vi "gugudan server.vi"() -> ()   [LabVIEW 2014]
panel:
  in  "사용설명서":bool
  out "로그인":bool
  in  "ID":string="ID"
  in  "PW":string="PW"
  in  "명령전달":bool
  in  "address":string="ip address"
  out "명령코드":i16[](array[numeric])
  out "참 거짓":string="상태창입니다."
  out "문자열":string="명령창 입니다."
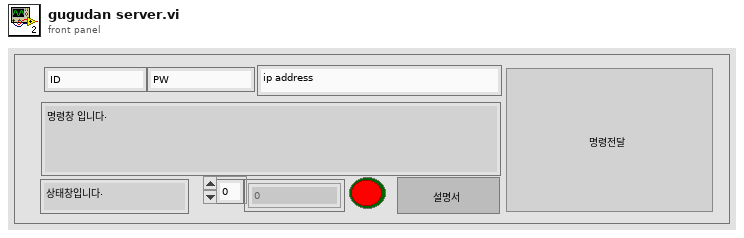
[diagram p1: front panel]
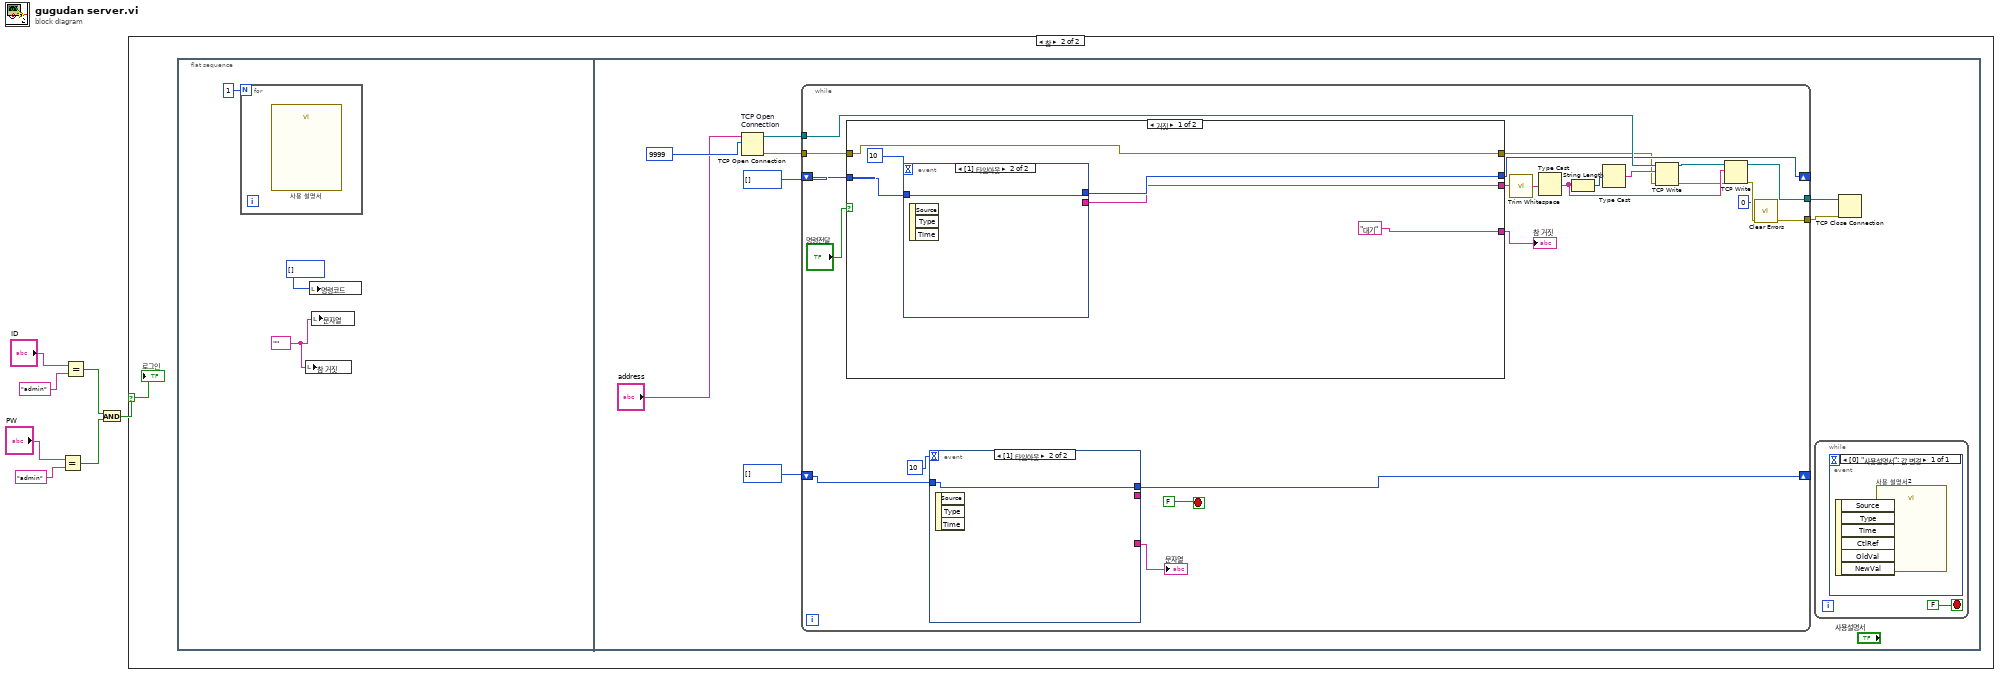
[diagram p0: block diagram]
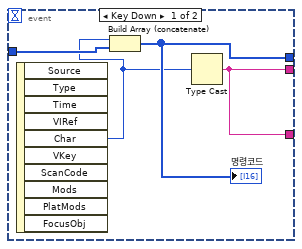
[diagram p3: hidden frame]
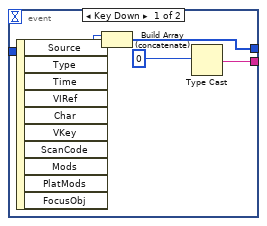
[diagram p4: hidden frame]
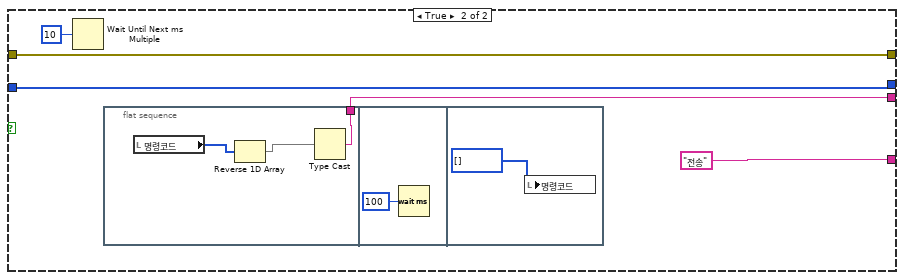
[diagram p5: hidden frame]
diagram:
  n1 = Equal?(x="PW", y="admin") -> (x = y?=w2:bool)
  n2 = Equal?(x="ID", y="admin") -> (x = y?=w3:bool)
  n3 = And(x=w3, y=w2) -> (x .and. y?=w1:bool)
  n4 = case shown="참" w1 {
    selector: w1 -> [_ w8]
    frame False {
    }
    frame True {
      n5 = flat-sequence {
        frame #0 {
          w10 = ""
          n6 = for {
            N: 1 -> [_]
            n7 = call "사용 설명서"() -> ()  [unwired: 10 in, 2 out]
          }
          n8 = local write "참 거짓"(w10) -> ()
          n9 = local write "명령코드"(i16[] []) -> ()
          n10 = local write "문자열"(w10) -> ()
        }
        frame #1 {
          n11 = TCP Open Connection "TCP Open \nConnection"(address="address", remote port or service name=u16 9999) -> (connection ID=w19:refnum<k5>, error out=w14:errorcluster)  [unwired: 3 in]
          n12 = while {
            tunnel: w19 -> [w41]
            tunnel: [w43] -> w17
            shift-right: [w32] -> _
            shift-left: i16[] [] -> [w42]
            shift-right: [w33] -> _
            shift-left: i16[] [] -> [w34]
            tunnel: w14 -> [w31]
            tunnel: [w23] -> w13
            stop <- FALSE stop-if-true
            n13 = case shown="거짓" "명령전달" {
              tunnel: w42 -> [w54 w65]
              tunnel: [w53 w65] -> w32
              tunnel: [w51 w61] -> w27
              tunnel: w31 -> [w50 w63]
              tunnel: [w50 w63] -> w30
              tunnel: ["대기" "전송"] -> w26
              frame False {
                n14 = event shown="[1] 타임아웃" {
                  selector: _ -> [_ _]
                  dyn-events: _ -> [_ _]
                  timeout: 10 -> [_ _]
                  tunnel: [w58 w60] -> w53
                  tunnel: w54 -> [w59 w60]
                  tunnel: [w56 _] -> w51
                  event Key Down {
                    n15 = event-data() -> ("Char"=w57:i16)  [unwired: 1 in, 9 out]
                    n16 = Build Array (concatenate)(w57, w59) -> (w58:i16[])
                    n17 = Type Cast(x=0) -> (*(type *) &x=w56:string)  [unwired: 1 in]
                  }
                  event Timeout {
                    n18 = event-data() -> ()  [unwired: 1 in, 3 out]
                  }
                }
              }
              frame True {
                n19 = Wait Until Next ms Multiple(millisecond multiple=u32 10) -> ()  [unwired: 1 out]
                n20 = flat-sequence {
                  tunnel: [w67] -> w61
                  frame #0 {
                    n21 = local read "명령코드"() -> (w68:i16[])
                    n22 = Reverse 1D Array(array=w68) -> (reversed array=w66:i16[])
                    n23 = Type Cast(x=w66) -> (*(type *) &x=w67:string)  [unwired: 1 in]
                  }
                  frame #1 {
                    n24 = Wait (ms)(milliseconds to wait=u32 100 ("대기 시간(ms)")) -> ()  [unwired: 1 out]
                  }
                  frame #2 {
                    n25 = local write "명령코드"(i16[] []) -> ()
                  }
                }
              }
            }
            "참 거짓" <- w26
            n26 = event shown="[1] 타임아웃" {
              selector: _ -> [_ _]
              dyn-events: _ -> [_ _]
              timeout: 10 -> [_ _]
              tunnel: [w45 w48] -> w33
              tunnel: [w47 _] -> w35
              tunnel: [w47 _] -> _
              tunnel: w34 -> [w46 w48]
              event Key Down {
                n27 = event-data() -> ("Char"=w44:i16)  [unwired: 1 in, 9 out]
                n28 = Build Array (concatenate)(w44, w46) -> (w45:i16[])
                "명령코드" <- w45
                n29 = Type Cast(x=w44) -> (*(type *) &x=w47:string)  [unwired: 1 in]
              }
              event Timeout {
                n30 = event-data() -> ()  [unwired: 1 in, 3 out]
              }
            }
            "문자열" <- w35
            n31 = call <vilib>:"Trim Whitespace.vi"("string"=w27) -> ("trimmed string"=w28:string)  [unwired: 1 in]
            n32 = Type Cast(x=w28) -> (*(type *) &x=w37:string)  [unwired: 1 in]
            n33 = String Length(string=w37) -> (length=w38:i32)
            n34 = Type Cast(x=w38) -> (*(type *) &x=w39:string)  [unwired: 1 in]
            n35 = TCP Write(connection ID=w41, data in=w39, error in (no error)=w30) -> (connection ID out=w40:refnum<k5>, error out=w29:errorcluster)  [unwired: 1 in, 1 out]
            n36 = TCP Write(connection ID=w40, data in=w37, error in (no error)=w29) -> (connection ID out=w43:refnum<k5>, error out=w22:errorcluster)  [unwired: 1 in, 1 out]
            n37 = call <vilib>:"Clear Errors.vi"("error in (no error)"=w22, "specific error code to clear (0: all)"=0) -> ("error out"=w23:errorcluster)  [unwired: 4 in, 1 out]
          }
          n38 = while {
            stop <- FALSE stop-if-true
            n39 = event shown="[0] \"사용설명서\": 값 변경" {
              selector: _ -> [_]
              dyn-events: _ -> [_]
              timeout: _ -> [_]
              event "사용설명서": Value Change {
                n40 = event-data() -> ()  [unwired: 1 in, 6 out]
                n41 = call "사용 설명서2"() -> ()  [unwired: 10 in, 2 out]
              }
            }
          }
          n42 = TCP Close Connection(connection ID=w17, error in (no error)=w13) -> ()  [unwired: 1 in, 2 out]
        }
      }
      "로그인" <- w8
    }
  }
